vi "DFD NStage MRate Filtering with State (Array).vi"(6 "state in":cluster{"state ":dbl[]}[](array[cluster]), 8 "error in (no error)":errorcluster, 10 "multirate filters":T1[](array[typedef]) {"mMRate_SumWl" min=1 max=32 step=1; "mMRate_InputIwl" min=1 max=32 step=1; "mMRate_GainWl" min=1 max=32 step=1; "mMRate_OutputWl" min=1 max=32 step=1; "mMRate_InputWl" min=1 max=32 step=1; "mMRate_CoefWl" min=1 max=32 step=1; "mMRate_Mode" items=["Default"=-1, "No Rate Change"=0, "Interpolation"=1, "Decimation"=2, "Interpolated"=3, "Rational"=4]}, 11 "signal in":dbl[](array[numeric])) -> (0 "error out":errorcluster, 3 "signal out":dbl[](array[numeric]), 4 "state out":cluster{"state ":dbl[]}[](array[cluster]))   [LabVIEW 2017, in "NI_DigFilterLicensed.lvlib"]
doc: "Filters a signal with a multistage multirate filter. You must specify the initial internal states in <B>state in</B> to filter the samples accurately. Wire data to the <B>signal in</B> input to determine the polymorphic instance to use or manually select the instance."
uses:
  <vilib>/addons/Digital Filter Design/NI_DigFilterLicensed.lvlib
  <vilib>/addons/Digital Filter Design/_Objects.llb/DFD Multirate Filter Obj.ctl
  <vilib>/addons/Digital Filter Design/_Objects.llb/DFD Multirate Mode.ctl
  <vilib>/addons/Digital Filter Design/_Objects.llb/DFD Coef Norm Type.ctl
  <vilib>/addons/Digital Filter Design/_Objects.llb/DFD Round-off Mode.ctl
  <vilib>/addons/Digital Filter Design/_Objects.llb/DFD FXP MRate Multiply Mode.ctl
  <vilib>/addons/Digital Filter Design/NI_DigFilter_Process.lvlib
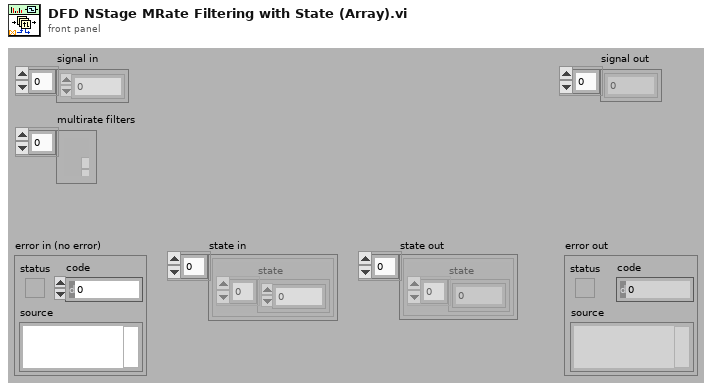
[diagram p1: front panel]
types:
  T1 = typedef "NI_DigFilterLicensed.lvlib/DFD Multirate Filter Obj.ctl" = cluster{"mMRate_Structure":enum16{"CIC", "FIR", "IIR", "Lattice"}, "mMRate_Mode":T2, "mMRate_Factor":i32, "mMRate_FIRParams":cluster{"mMRate_FIR_H":dbl[], "mMRate_FIR_IsNyquist?":bool, "mMRate_FIR_IsSymmetric?":bool}, "mMRate_CICParams":cluster{"mMRate_CIC_#Stage":i32, "mMRate_CIC_Lag":i32, "mMRate_CIC_Type":enum16{"Lowpass", "Highpass"}}, "mMRate_Order":i32, "mMRate_Version":string, "mMRate_Comments":string, "mMRate_RationalFactor":cluster{"mMRate_L":i32, "mMRate_M":i32}, "mMRate_Fs":dbl, "mMRate_Quantized?":bool, "mMRate_QFilterGain":dbl, "mMRate_CoefWl":i16, "mMRate_Scaling":cluster{"mMRate_ScaleByPowerOf2?":bool, "mMRate_ScaleType":T3}, "mMRate_InputWl":i16, "mMRate_OutputWl":i16, "mMRate_OutputMode":T4, "mMRate_MultMode":T5, "mMRate_BitPruning":bool, "mMRate_GainWl":i16, "mMRate_OutputFwl":i16, "mMRate_SumIwl":i16, "mMRate_InputIwl ":i16, "mMRate_SumWl":i16, "mMRate_CoefIwl":i16}
  T2 = typedef "NI_DigFilterLicensed.lvlib/DFD Multirate Mode.ctl" = i16
  T3 = typedef "NI_DigFilterLicensed.lvlib/DFD Coef Norm Type.ctl" = enum16{"No Norm", "Time Domain 1-Norm", "Time Domain 2-Norm", "Time Domain Inf-Norm"}
  T4 = typedef "NI_DigFilterLicensed.lvlib/DFD Round-off Mode.ctl" = enum16{"Nearest", "Truncation"}
  T5 = typedef "NI_DigFilterLicensed.lvlib/DFD FXP MRate Multiply Mode.ctl" = enum16{"Truncated", "Full"}
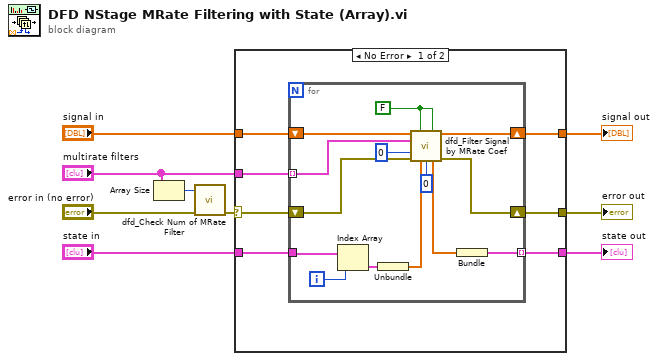
[diagram p0: block diagram]
diagram:
  n1 = Array Size(array="multirate filters") -> (size(s)=w1:i32)
  n2 = call <vilib>:"dfd_Check Num of MRate Filter.vi"("error in (no error)"="error in (no error)", "#MRate in"=w1) -> ("error out"=w2:errorcluster)  [unwired: 9 out]
  n3 = case shown="No Error" w2 {
    selector: w2 -> [w10 w31]
    tunnel: [w14 w31] -> w9
    tunnel: "multirate filters" -> [w15 _]
    tunnel: "signal in" -> [w12 _]
    tunnel: [w16 _] -> w7
    tunnel: "state in" -> [w13 _]
    tunnel: [w11 _] -> w5
    frame No Error {
      n4 = for {
        tunnel: w15 -> [w21] mode=indexing
        tunnel: [w30] -> w11 mode=indexing
        tunnel: w13 -> [w29]
        shift-right: [w22] -> w16
        shift-left: w12 -> [w23]
        shift-right: [w19] -> w14
        shift-left: w10 -> [w20]
        i -> [w28]
        w24 = FALSE ("initH?")
        n5 = Index Array(array=w29, index=w28) -> (element=w27:cluster{"state ":dbl[]})
        n6 = Unbundle(w27) -> ("state"=w18:dbl[])
        n7 = call <vilib>:"dfd_Filter Signal by MRate Coef.vi"("signal in"=w23, "initH?"=w24, "zeroPhaseH?"=w24, "multirate filter"=w21, "skipPoint In"=0, "error in (no error)"=w20, "state in"=w18, "outputPhase"=0) -> ("signal out"=w22:dbl[], "state out"=w17:dbl[], "error out"=w19:errorcluster)  [unwired: 5 out]
        n8 = Bundle("state out"=w17) -> (w30:cluster{"state out":dbl[]})  [unwired: 1 in]
      }
    }
    frame Error {
    }
  }
  "error out" <- w9
  "signal out" <- w7
  "state out" <- w5
